vi "Event Log.Create.vi"(6 "Working Dirs":T1, 7 "Ping Check":bool=TRUE, 8 "Error In":errorcluster, 11 "Q In":refnum<queue>) -> (0 "Error Out":errorcluster, 1 "Name Out":string, 3 "reference out":refnum<vi>)   [LabVIEW 2024, in "EQMF.lvlib" / "Event Log.lvlib"]
uses:
  Event Log.lvlib
  Queues/Q.Element.ctl
  Module/Module.Working Dirs.ctl
  _Core/Event Log.vi
  Module/Module Utils.lvlib
  Queues/Queue Utils.lvlib
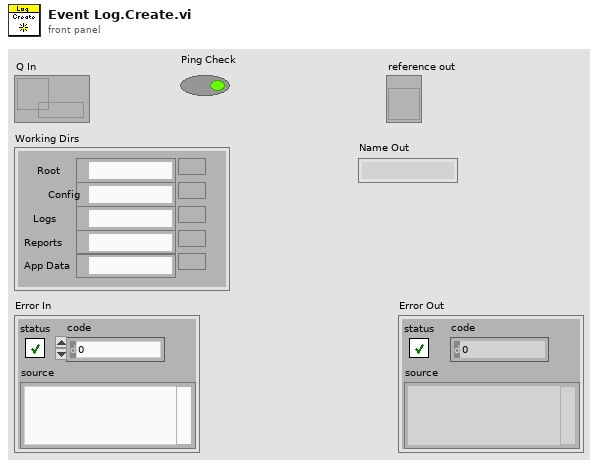
[diagram p1: front panel]
types:
  T1 = typedef "EQMF.lvlib/Module Utils.lvlib/Module.Working Dirs.ctl" = cluster{"Root":path, "Config":path, "Logs":path, "Reports":path, "App Data":path}
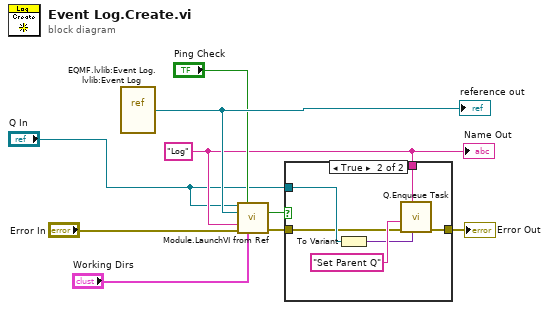
[diagram p0: block diagram]
diagram:
  w5 = "Log" ("Name [Do not use!]")
  n1 = vi-ref "EQMF.lvlib:Event Log.lvlib:Event Log.vi"() -> (w8:refnum<vi>)
  "reference out" <- w8
  n2 = call "Module.LaunchVI from Ref.vi"("Parent Q"="Q In", "Ping Check"="Ping Check", "VI Ref In"=w8, "Q Name"=w5, "error in"="Error In", "Working Dirs"="Working Dirs") -> ("Already Exists"=w1:bool, "error out"=w2:errorcluster)  [unwired: 7 in, 1 out]
  n3 = case shown="True" w1 {
    tunnel: w5 -> [_ w15]
    tunnel: "Q In" -> [_ w14]
    tunnel: [w10 w12] -> w3
    tunnel: w2 -> [w10 w11]
    frame False {
    }
    frame True {
      n4 = To Variant(anything=w14) -> (Variant=w13:variant)
      n5 = call "Q.Enqueue Task.vi"("Data1"=w13, "Q Name"=w15, "Error In"=w11, "Task Name"="Set Parent Q") -> ("error out"=w12:errorcluster)  [unwired: 6 in, 1 out]
    }
  }
  "Error Out" <- w3
  "Name Out" <- w5
